vi "Config Program.vi"(8 "error in (no error)":errorcluster, 11 "Prog in":T1) -> (0 "error out":errorcluster, 3 "Prog out":T1)   [LabVIEW 2014, in "SeqLoop.lvlib"]
doc: "Configura un Programa que contiene la secuencias de autocero, ciclo y especiales."
uses:
  SeqLoop.lvlib
  TypeDefs/Program.ctl
  Classes/STEP/STEP.lvclass
  TypeDefs/Sequence.ctl
  TypeDefs/LogicParsedExpression.ctl
panel:
  in  "Total Meds. Aux.:":i32
  in  "Total Meds.:":i32
  out "Tipo de Programa":string
  in  "Config Special":bool
  in  "Save":bool
  in  "Close":bool
  in  "Config AutoZero":bool
  in  "Diseño":string
  in  "Cód. Prog.":i32
  in  "Autor":string
  in  "Nombre Programa":string
  in  "Descripción":string
  in  "Pieza":i32
  in  "Operación":i32
  in  "Config Measurement":bool
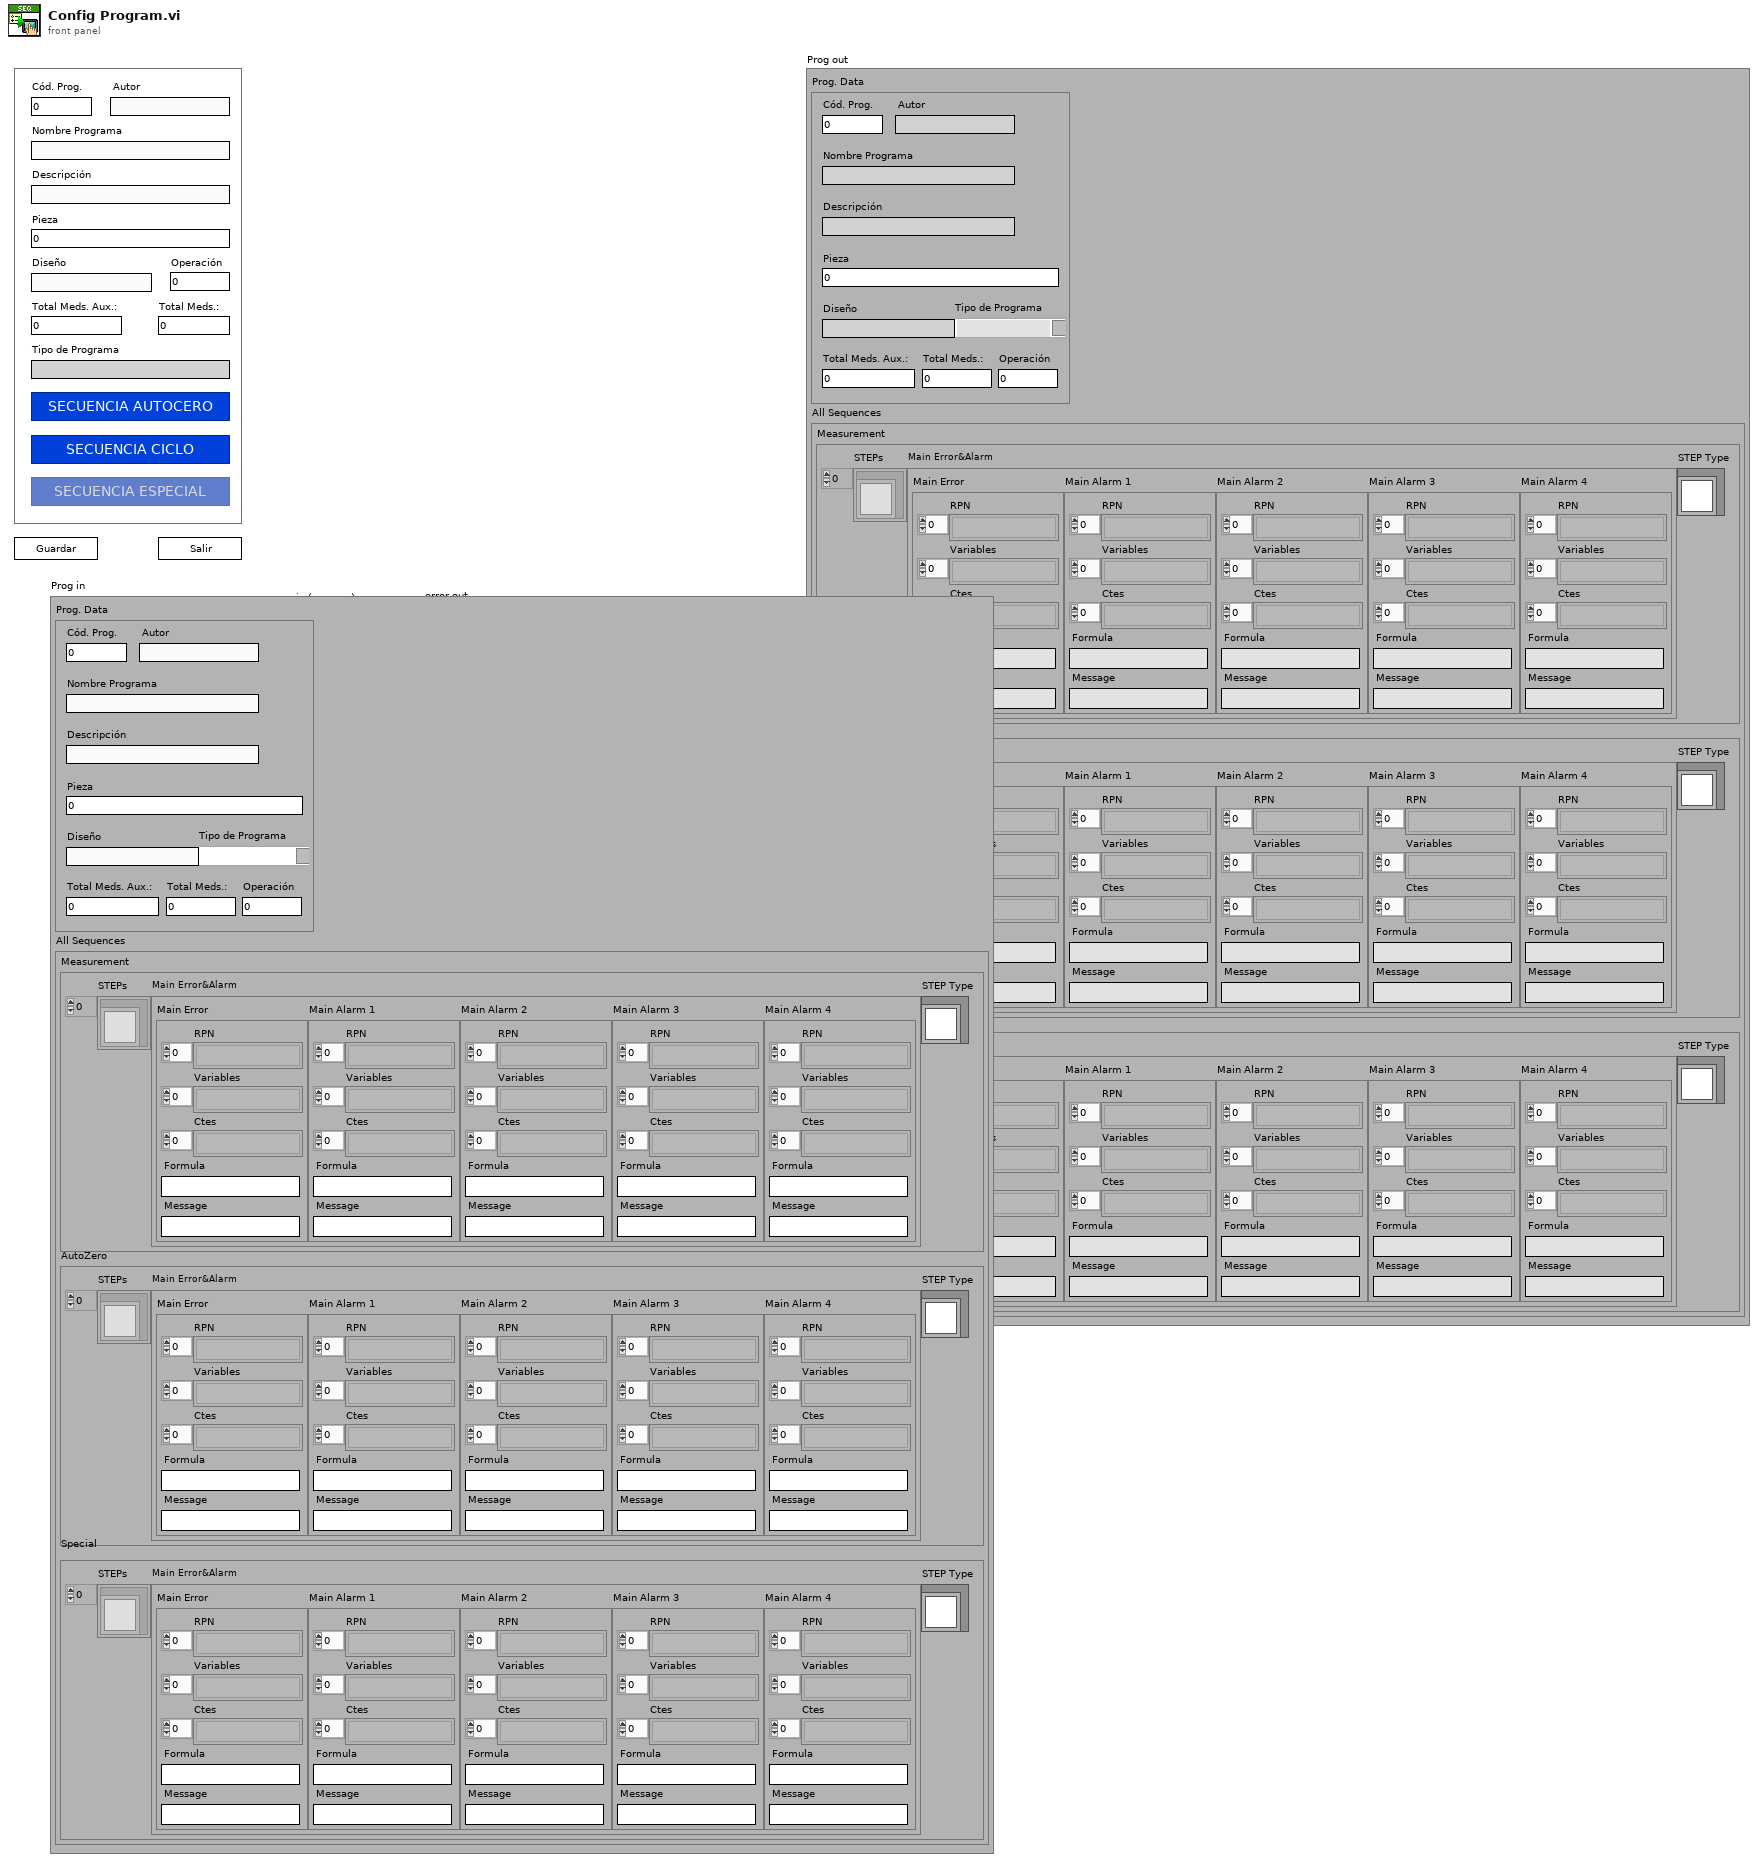
[diagram p1: front panel]
types:
  T1 = typedef "SeqLoop.lvlib/Program.ctl" = cluster{"Prog. Data":cluster{"Tipo de Programa":string, "Operación":i32, "Pieza":i32, "Descripción":string, "Nombre Programa":string, "Autor":string, "Cód. Prog.":i32, "Diseño":string, "Total Meds.:":i32, "Total Meds. Aux.:":i32}, "All Sequences":cluster{"Measurement":T2, "AutoZero":T2, "Special":T2}}
  T2 = typedef "SeqLoop.lvlib/Sequence.ctl" = cluster{"STEPs":refnum<class "STEP.lvclass">[], "Main Error&Alarm":cluster{"Main Error":T3, "Main Alarm 1":T3, "Main Alarm 2":T3, "Main Alarm 3":T3, "Main Alarm 4":T3}, "STEP Type":refnum<class "STEP.lvclass">}
  T3 = typedef "SeqLoop.lvlib/LogicParsedExpression.ctl" = cluster{"RPN ":string[], "Variables":string[], "Ctes":string[], "Formula":string, "Message":string}
  T4 = enum8{"Enabled", "Disabled", "Disabled and Grayed Out"}
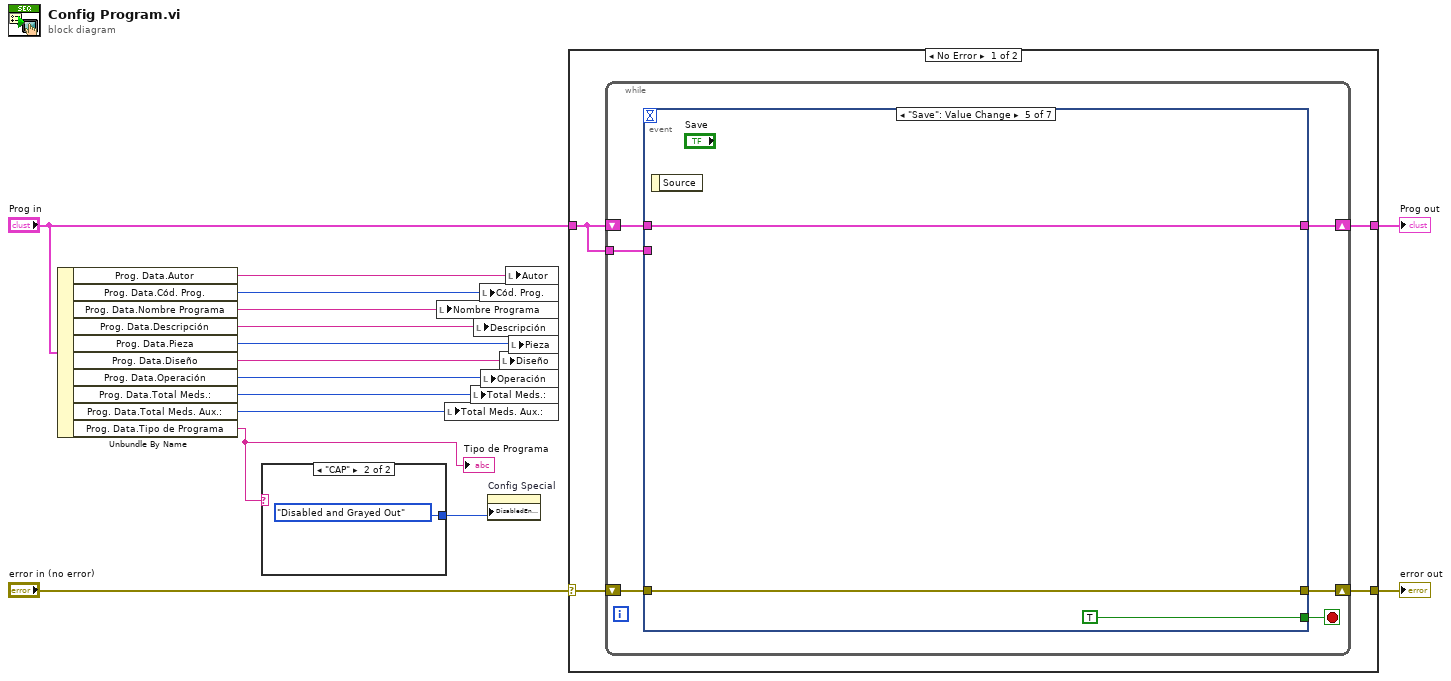
[diagram p0: block diagram]
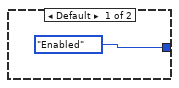
[diagram p2: hidden frame]
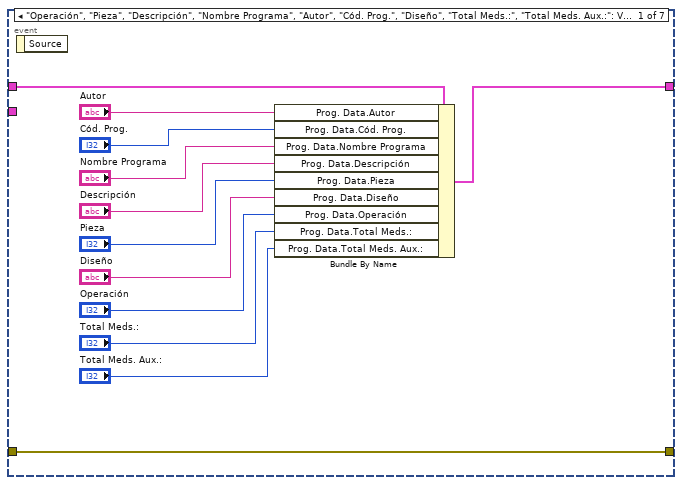
[diagram p3: hidden frame]
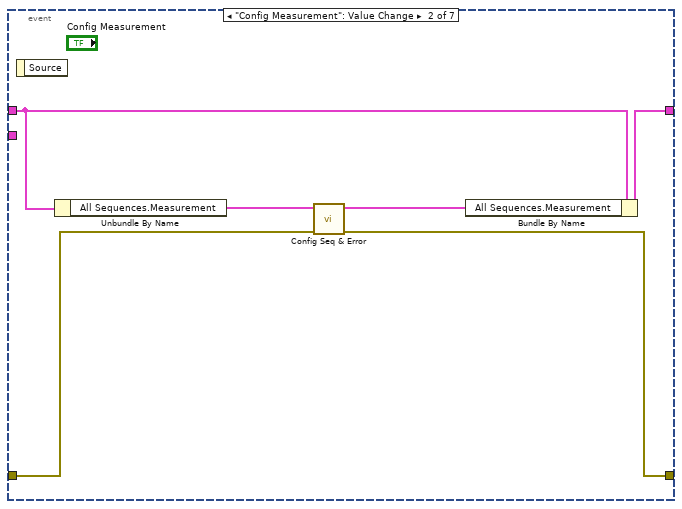
[diagram p4: hidden frame]
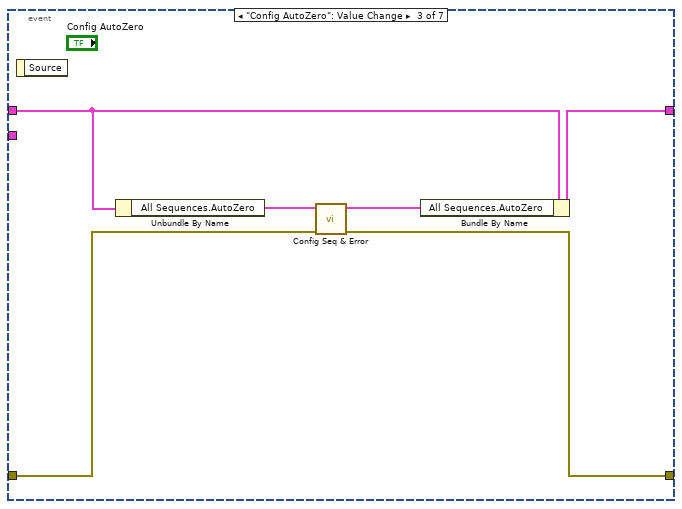
[diagram p5: hidden frame]
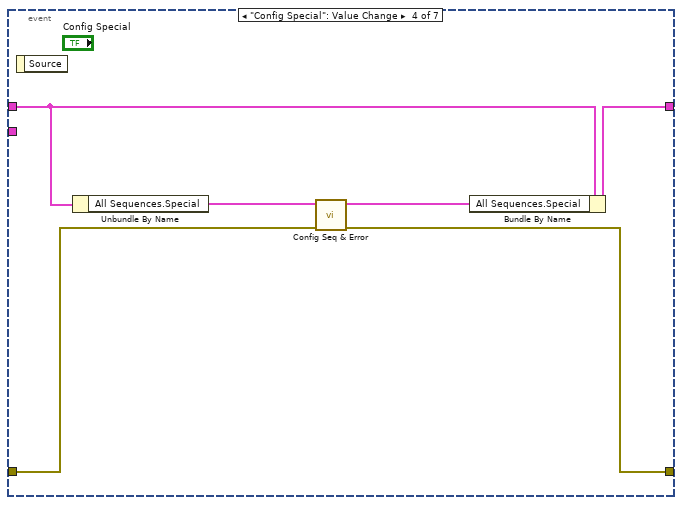
[diagram p6: hidden frame]
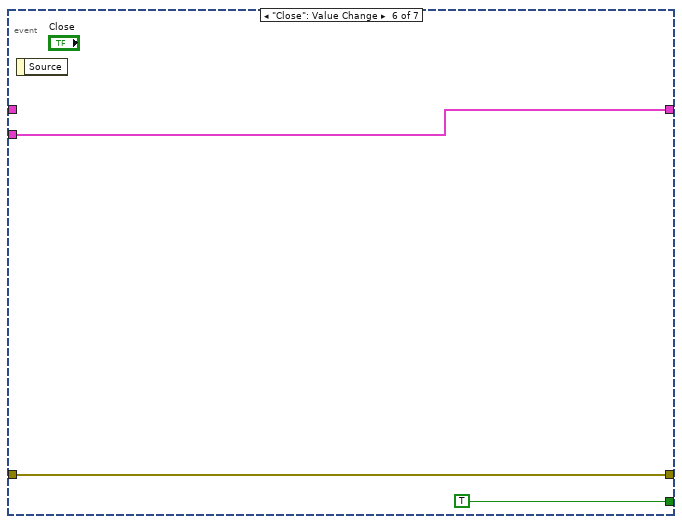
[diagram p7: hidden frame]
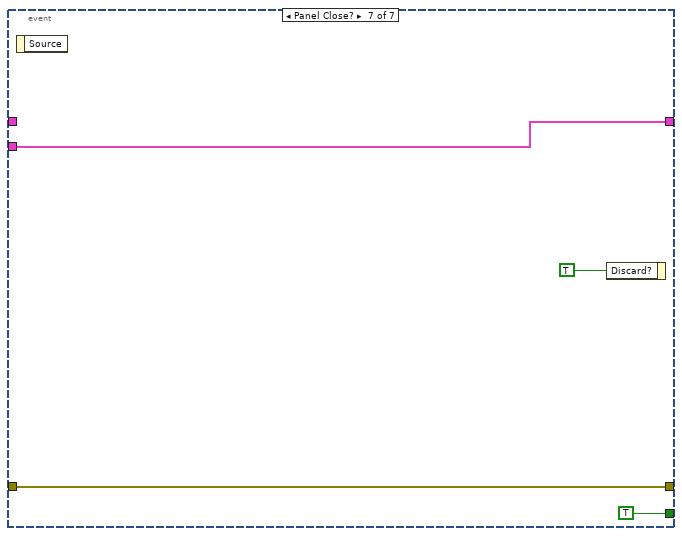
[diagram p8: hidden frame]
diagram:
  n1 = Unbundle By Name("Prog in") -> ("Prog. Data.Autor"=w11:string, "Prog. Data.Cód. Prog."=w10:i32, "Prog. Data.Nombre Programa"=w9:string, "Prog. Data.Descripción"=w8:string, "Prog. Data.Pieza"=w7:i32, "Prog. Data.Diseño"=w6:string, "Prog. Data.Operación"=w5:i32, "Prog. Data.Total Meds.:"=w2:i32, "Prog. Data.Total Meds. Aux.:"=w1:i32, "Prog. Data.Tipo de Programa"=w3:string)
  "Tipo de Programa" <- w3
  n2 = case shown="\"CAP\"" w3 {
    tunnel: [T4."Enabled" ("Disabled") T4."Disabled and Grayed Out" ("Disabled")] -> w4
    frame Default {
    }
    frame "CAP" {
    }
  }
  n3 = local write "Nombre Programa"(w9) -> ()
  n4 = local write "Total Meds. Aux.:"(w1) -> ()
  n5 = local write "Total Meds.:"(w2) -> ()
  n6 = local write "Descripción"(w8) -> ()
  n7 = local write "Cód. Prog."(w10) -> ()
  n8 = local write "Operación"(w5) -> ()
  n9 = property on="Config Special" class="Bool"("DisabledEnum"=w4) -> ()  [unwired: 2 in, 2 out]
  n10 = local write "Diseño"(w6) -> ()
  n11 = local write "Autor"(w11) -> ()
  n12 = local write "Pieza"(w7) -> ()
  n13 = case shown="No Error" "error in (no error)" {
    selector: "error in (no error)" -> [w21 w69]
    tunnel: [w20 w69] -> w14
    tunnel: "Prog in" -> [w18 w68]
    tunnel: [w19 w68] -> w13
    frame No Error {
      n14 = while {
        shift-right: [w26] -> w20
        shift-left: w21 -> [w27]
        shift-right: [w24] -> w19
        shift-left: w18 -> [w25]
        tunnel: w18 -> [w22]
        stop <- w23 stop-if-true
        n15 = event shown="[4] \"Save\": Value Change" {
          selector: _ -> [_ _ _ _ _ _ _]
          dyn-events: _ -> [_ _ _ _ _ _ _]
          timeout: _ -> [_ _ _ _ _ _ _]
          tunnel: w27 -> [w39 w41 w46 w52 w59 w61 w66]
          tunnel: [w39 w40 w47 w53 w59 w61 w66] -> w26
          tunnel: w25 -> [w38 w45 w51 w57 w58 _ _]
          tunnel: [w37 w44 w50 w56 w58 w63 w64] -> w24
          tunnel: [_ _ _ _ TRUE TRUE TRUE] -> w23
          tunnel: w22 -> [_ _ _ _ _ w63 w64]
          event "Operación", "Pieza", "Descripción", "Nombre Programa", "Autor", "Cód. Prog.", "Diseño", "Total Meds.:", "Total Meds. Aux.:": Value Change {
            n16 = event-data() -> ()  [unwired: 1 in, 1 out]
            n17 = Bundle By Name(cluster=w38, "Prog. Data.Autor"="Autor", "Prog. Data.Cód. Prog."="Cód. Prog.", "Prog. Data.Nombre Programa"="Nombre Programa", "Prog. Data.Descripción"="Descripción", "Prog. Data.Pieza"="Pieza", "Prog. Data.Diseño"="Diseño", "Prog. Data.Operación"="Operación", "Prog. Data.Total Meds.:"="Total Meds.:", "Prog. Data.Total Meds. Aux.:"="Total Meds. Aux.:") -> (w37:T1)
          }
          event "Config Measurement": Value Change {
            n18 = event-data() -> ()  [unwired: 1 in, 1 out]
            n19 = Unbundle By Name(w45) -> ("All Sequences.Measurement"=w42:T2)
            n20 = call "Config Seq & Error.vi"("error in (no error)"=w41, "Sequences"=w42) -> ("error out"=w40:errorcluster, "Sequences"=w43:T2)  [unwired: 8 in]
            n21 = Bundle By Name(cluster=w45, "All Sequences.Measurement"=w43) -> (w44:T1)
          }
          event "Config AutoZero": Value Change {
            n22 = event-data() -> ()  [unwired: 1 in, 1 out]
            n23 = Unbundle By Name(w51) -> ("All Sequences.AutoZero"=w49:T2)
            n24 = call "Config Seq & Error.vi"("error in (no error)"=w46, "Sequences"=w49) -> ("error out"=w47:errorcluster, "Sequences"=w48:T2)  [unwired: 8 in]
            n25 = Bundle By Name(cluster=w51, "All Sequences.AutoZero"=w48) -> (w50:T1)
          }
          event "Config Special": Value Change {
            n26 = event-data() -> ()  [unwired: 1 in, 1 out]
            n27 = Unbundle By Name(w57) -> ("All Sequences.Special"=w55:T2)
            n28 = call "Config Seq & Error.vi"("error in (no error)"=w52, "Sequences"=w55) -> ("error out"=w53:errorcluster, "Sequences"=w54:T2)  [unwired: 8 in]
            n29 = Bundle By Name(cluster=w57, "All Sequences.Special"=w54) -> (w56:T1)
          }
          event "Save": Value Change {
            n30 = event-data() -> ()  [unwired: 1 in, 1 out]
          }
          event "Close": Value Change {
            n31 = event-data() -> ()  [unwired: 1 in, 1 out]
          }
          event Panel Close? {
            n32 = event-data() -> ()  [unwired: 1 in, 1 out]
            n33 = event-data("Discard?"=TRUE) -> ()  [unwired: 1 in, 1 out]
          }
        }
      }
    }
    frame Error {
    }
  }
  "error out" <- w14
  "Prog out" <- w13
